vi "OS_Get_An_Control_Index.vi"() -> (2 "Array":u16[](array[numeric]))   [LabVIEW 2016]
uses:
  <vilib>/Utility/file.llb/Read Delimited Spreadsheet (string).vi
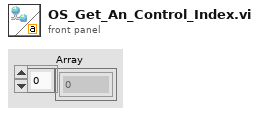
[diagram p1: front panel]
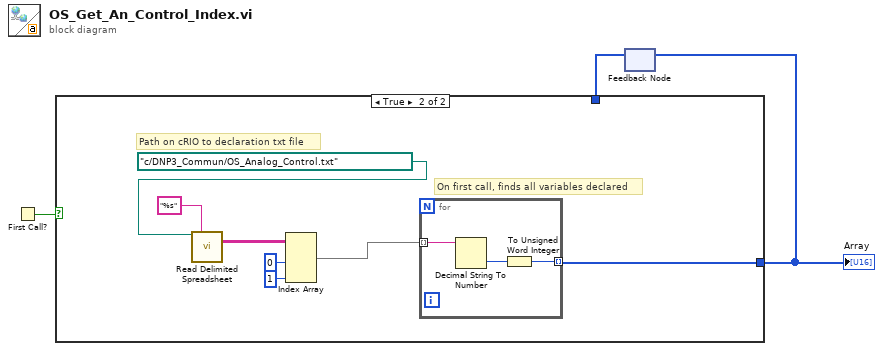
[diagram p0: block diagram]
diagram:
  n1 = First Call?() -> (First Call?: T/F=w3:bool)
  n2 = feedback #1() -> (w1:u16[])  [unwired: 1 in]
  n3 = case shown="True" w3 {
    tunnel: [w4 w5] -> w2
    tunnel: w1 -> [w4 _]
    frame False {
    }
    frame True {
      # "On first call, finds all variables declared"
      # "Path on cRIO to declaration txt file"
      n4 = call-poly <vilib>:"Read Delimited Spreadsheet.vi"("file path (dialog if empty)"=path "c:/DNP3_Commun/OS_Analog_Control.txt" ("file path (use dialog)"), "format (%s)"="%s") -> ("all rows"=w9:string[][])  [unwired: 8 in, 5 out]
      n5 = Index Array(array=w9, index (col) #1=0 ("disabled index (col)"), index (col) #2=1 ("index (col)")) -> (element #1=w6:string[])  [unwired: 2 in, 1 out]
      n6 = for {
        tunnel: [w14] -> w5 mode=indexing
        tunnel: w6 -> [w12] mode=indexing
        n7 = Decimal String To Number(string=w12) -> (number=w13:i32)  [unwired: 2 in, 1 out]
        n8 = To Unsigned Word Integer(number=w13) -> (unsigned 16bit integer=w14:u16)
      }
    }
  }
  "Array" <- w2
  n9 = feedback-in #1(w2) -> ()
